vi "DMSO_EC_reload_MQ_NaCl_subVI.vi"(6 "COM Port":refnum<visa-resource-name>="COM7", 7 "Pump Parameters":T1={"Speed 1"="100", "Speed 2"="250", "Speed 3"="250", "Speed 4"="250", "UW/Sample"="5", "Sparge"="2", "Std"="4", "Waste"="15", "Air"="14", "Milli-Q"="1", "H2SO4"="6", "NaOH"="3", "Catalyst"="7", "Cell (H+ side)"="8", "Cell (sample side)"="9", "NaCl"="9"}, 8 "step to ml":dbl=1920.0, 10 "Sample Vol. (mL)":dbl, 11 "Extra Milli-Q (ml)":dbl=4.0) -> ()   [LabVIEW 2021]
panel:
  out "Full Command":string="V100O1P7680O9D7680"
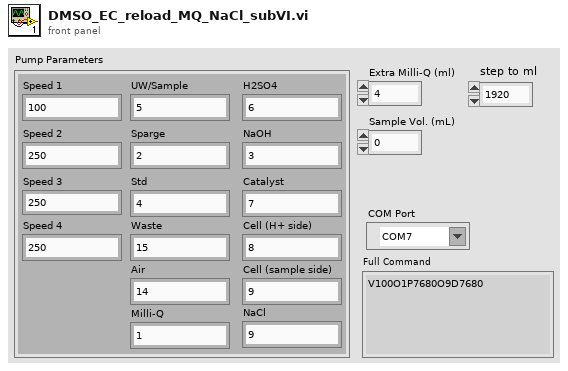
[diagram p1: front panel]
types:
  T1 = cluster{"Speed 1":string, "Speed 2":string, "Speed 3":string, "Speed 4":string, "UW/Sample":string, "Sparge":string, "Std":string, "Waste":string, "Air":string, "Milli-Q":string, "H2SO4":string, "NaOH":string, "Catalyst":string, "Cell (H+ side)":string, "Cell (sample side)":string, "NaCl":string}
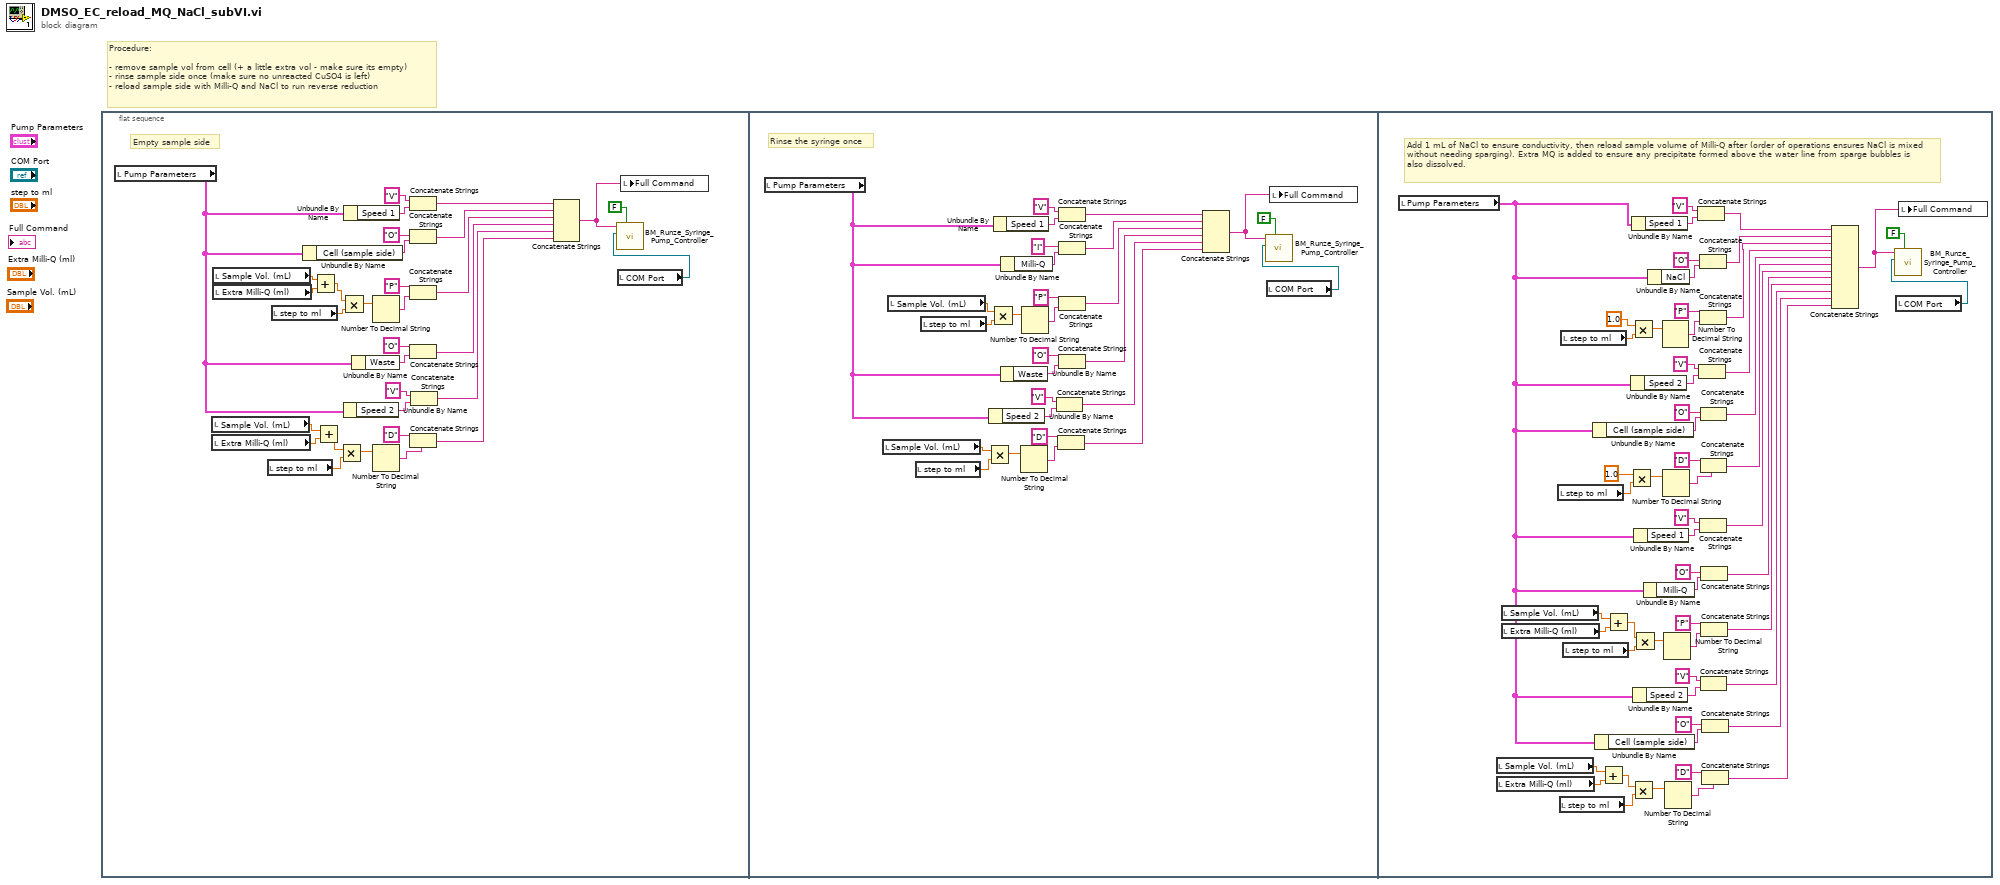
[diagram p0: block diagram]
diagram:
  # "Procedure:\n\n- remove sample vol from cell (+ a little extra vol - make sure its empty)\n- rinse sample side once (make sure no unreacted CuSO4 is left)\n- reload sample side with Milli-Q and NaCl to run reverse reduction"
  n1 = flat-sequence {
    frame #0 {
      # "Empty sample side"
      n2 = local read "Pump Parameters"() -> (w10:T1)
      n3 = local read "Sample Vol. (mL)"() -> (w3:dbl)
      n4 = local read "Extra Milli-Q (ml)"() -> (w2:dbl)
      n5 = local read "Sample Vol. (mL)"() -> (w6:dbl)
      n6 = local read "Extra Milli-Q (ml)"() -> (w5:dbl)
      n7 = local read "step to ml"() -> (w23:dbl)
      n8 = local read "step to ml"() -> (w28:dbl)
      n9 = Unbundle By Name(w10) -> ("Cell (sample side)"=w8:string)
      n10 = Add(x=w6, y=w5) -> (x+y=w4:dbl)
      n11 = Add(x=w3, y=w2) -> (x+y=w1:dbl)
      n12 = Multiply(x=w1, y=w23) -> (x*y=w24:dbl)
      n13 = Multiply(x=w4, y=w28) -> (x*y=w29:dbl)
      n14 = Unbundle By Name(w10) -> ("Speed 2"=w13:string)
      n15 = Unbundle By Name(w10) -> ("Speed 1"=w30:string)
      n16 = Unbundle By Name(w10) -> ("Waste"=w7:string)
      n17 = Number To Decimal String(number=w29) -> (decimal integer string=w26:string)  [unwired: 1 out]
      n18 = Number To Decimal String(number=w24) -> (decimal integer string=w21:string)  [unwired: 1 out]
      n19 = Concatenate Strings("V", w30) -> (w20:string)
      n20 = Concatenate Strings("O", w8) -> (w19:string)
      n21 = Concatenate Strings("P", w26) -> (w18:string)
      n22 = Concatenate Strings("O", w7) -> (w17:string)
      n23 = Concatenate Strings("D", w21) -> (w11:string)
      n24 = Concatenate Strings("V", w13) -> (w12:string)
      n25 = Concatenate Strings(w20, w19, w18, w17, w12, w11) -> (w16:string)
      n26 = local read "COM Port"() -> (w15:refnum<visa-resource-name>)
      n27 = call "BM_Runze_Syringe_Pump_Controller.vi"("Initialize Plunger?"=FALSE ("Initialize?"), "COM Port (Runze)"=w15, "Enter Command"=w16) -> ()  [unwired: 6 in, 3 out]
      n28 = local write "Full Command"(w16) -> ()
    }
    frame #1 {
      # "Rinse the syringe once"
      n29 = local read "Pump Parameters"() -> (w33:T1)
      n30 = local read "Sample Vol. (mL)"() -> (w43:dbl)
      n31 = local read "Sample Vol. (mL)"() -> (w47:dbl)
      n32 = local read "step to ml"() -> (w41:dbl)
      n33 = local read "step to ml"() -> (w52:dbl)
      n34 = Multiply(x=w43, y=w41) -> (x*y=w42:dbl)
      n35 = Unbundle By Name(w33) -> ("Speed 2"=w37:string)
      n36 = Multiply(x=w47, y=w52) -> (x*y=w51:dbl)
      n37 = Unbundle By Name(w33) -> ("Speed 1"=w50:string)
      n38 = Unbundle By Name(w33) -> ("Waste"=w44:string)
      n39 = Unbundle By Name(w33) -> ("Milli-Q"=w46:string)
      n40 = Number To Decimal String(number=w42) -> (decimal integer string=w39:string)  [unwired: 1 out]
      n41 = Number To Decimal String(number=w51) -> (decimal integer string=w54:string)  [unwired: 1 out]
      n42 = Concatenate Strings("V", w37) -> (w35:string)
      n43 = Concatenate Strings("D", w39) -> (w34:string)
      n44 = Concatenate Strings("V", w50) -> (w55:string)
      n45 = Concatenate Strings("I", w46) -> (w56:string)
      n46 = Concatenate Strings("P", w54) -> (w57:string)
      n47 = Concatenate Strings("O", w44) -> (w36:string)
      n48 = Concatenate Strings(w55, w56, w57, w36, w35, w34) -> (w58:string)
      n49 = local read "COM Port"() -> (w59:refnum<visa-resource-name>)
      n50 = call "BM_Runze_Syringe_Pump_Controller.vi"("Initialize Plunger?"=FALSE ("Initialize?"), "COM Port (Runze)"=w59, "Enter Command"=w58) -> ()  [unwired: 6 in, 3 out]
      n51 = local write "Full Command"(w58) -> ()
    }
    frame #2 {
      # "Add 1 mL of NaCl to ensure conductivity, then reload sample volume of Milli-Q after (order of operations ensures NaCl is mixed without needing sparging). Extra MQ is added to ensure any precipitate formed above the water line from sparge bubbles is also dissolved."
      n52 = local read "Pump Parameters"() -> (w79:T1)
      n53 = local read "Sample Vol. (mL)"() -> (w63:dbl)
      n54 = local read "Extra Milli-Q (ml)"() -> (w64:dbl)
      n55 = local read "Sample Vol. (mL)"() -> (w66:dbl)
      n56 = local read "Extra Milli-Q (ml)"() -> (w65:dbl)
      n57 = local read "step to ml"() -> (w104:dbl)
      n58 = local read "step to ml"() -> (w95:dbl)
      n59 = local read "step to ml"() -> (w111:dbl)
      n60 = local read "step to ml"() -> (w88:dbl)
      n61 = Unbundle By Name(w79) -> ("Cell (sample side)"=w106:string)
      n62 = Unbundle By Name(w79) -> ("Cell (sample side)"=w93:string)
      n63 = Add(x=w63, y=w64) -> (x+y=w61:dbl)
      n64 = Add(x=w66, y=w65) -> (x+y=w62:dbl)
      n65 = Multiply(x=1.0, y=w104) -> (x*y=w105:dbl)
      n66 = Multiply(x=1.0, y=w111) -> (x*y=w112:dbl)
      n67 = Multiply(x=w61, y=w95) -> (x*y=w94:dbl)
      n68 = Unbundle By Name(w79) -> ("Speed 2"=w100:string)
      n69 = Unbundle By Name(w79) -> ("Speed 1"=w108:string)
      n70 = Multiply(x=w62, y=w88) -> (x*y=w87:dbl)
      n71 = Unbundle By Name(w79) -> ("Speed 2"=w99:string)
      n72 = Unbundle By Name(w79) -> ("Speed 1"=w91:string)
      n73 = Unbundle By Name(w79) -> ("Milli-Q"=w85:string)
      n74 = Unbundle By Name(w79) -> ("NaCl"=w115:string)
      n75 = Number To Decimal String(number=w112) -> (decimal integer string=w109:string)  [unwired: 1 out]
      n76 = Number To Decimal String(number=w105) -> (decimal integer string=w102:string)  [unwired: 1 out]
      n77 = Number To Decimal String(number=w87) -> (decimal integer string=w90:string)  [unwired: 1 out]
      n78 = Number To Decimal String(number=w94) -> (decimal integer string=w97:string)  [unwired: 1 out]
      n79 = Concatenate Strings("V", w108) -> (w78:string)
      n80 = Concatenate Strings("V", w100) -> (w75:string)
      n81 = Concatenate Strings("O", w115) -> (w77:string)
      n82 = Concatenate Strings("P", w109) -> (w76:string)
      n83 = Concatenate Strings("V", w91) -> (w72:string)
      n84 = Concatenate Strings("O", w106) -> (w74:string)
      n85 = Concatenate Strings("D", w102) -> (w73:string)
      n86 = Concatenate Strings("V", w99) -> (w69:string)
      n87 = Concatenate Strings("O", w85) -> (w71:string)
      n88 = Concatenate Strings("P", w90) -> (w70:string)
      n89 = Concatenate Strings("O", w93) -> (w68:string)
      n90 = Concatenate Strings("D", w97) -> (w67:string)
      n91 = Concatenate Strings(w78, w77, w76, w75, w74, w73, w72, w71, w70, w69, w68, w67) -> (w84:string)
      n92 = local read "COM Port"() -> (w83:refnum<visa-resource-name>)
      n93 = call "BM_Runze_Syringe_Pump_Controller.vi"("Initialize Plunger?"=FALSE ("Initialize?"), "COM Port (Runze)"=w83, "Enter Command"=w84) -> ()  [unwired: 6 in, 3 out]
      n94 = local write "Full Command"(w84) -> ()
    }
  }
